vi "PQ_Windowed RMS.vi"(10 "data":waveform(dbl)[](array[waveform])) -> (1 "Resampled Data":dbl[][](graph), 2 "RMS":dbl[][](graph))   [LabVIEW 2014]
uses:
  <vilib>/Analysis/2dsp.llb/Rational Resample (multi-channel, DBL).vi
  <vilib>/imath/engines/lvmath2/RunTimeEngine/BuiltInFunctions/length/NIMS_length(GV).vi
  <instcachedir>/0/NIMS_length(GV)_08A3D13377FD4E4B96F5795FBF3698FA.lvgen/NIMS_length(GV)_08A3D13377FD4E4B96F5795FBF3698FA_000.vi
  <vilib>/imath/engines/lvmath2/RunTimeEngine/CommandStatement/MC_CommandStatement_break.vi
  <vilib>/imath/engines/lvmath2/RunTimeEngine/RangeToken/NIMS_Range.vi
  <instcachedir>/0/NIMS_Range_9BCE657718DF4976A877346C61F22738.lvgen/NIMS_Range_9BCE657718DF4976A877346C61F22738_000.vi
  <vilib>/imathl/engines/lvmath/Functions/Error Handling/Create Error.vi
  <vilib>/imath/engines/lvmath2/RunTimeEngine/VariableToken/NIMS_VariableToken_CondDefinedDefinedByReplace.vi
  <instcachedir>/0/NIMS_VariableToken_CondDefinedDefinedByReplace_D162CFFC24174562A9FEA619A91E1A56.lvgen/NIMS_VariableToken_CondDefinedDefinedByReplace_D162CFFC24174562A9FEA619A91E1A56_000.vi
  <vilib>/imath/engines/lvmath2/RunTimeSupport/NIMS_Error if Not Equal.vi
  <instcachedir>/0/NIMS_Error if Not Equal_8A0E9F659B9142D69417CC259581C4FD.lvgen/NIMS_Error if Not Equal_8A0E9F659B9142D69417CC259581C4FD_000.vi
  <instcachedir>/0/NIMS_Error if Not Equal_8A0E9F659B9142D69417CC259581C4FD.lvgen/NIMS_Error if Not Equal_8A0E9F659B9142D69417CC259581C4FD_001.vi
  <vilib>/imath/engines/lvmath2/RunTimeEngine/IndexRead/NIMS V(V).vi
  <instcachedir>/0/NIMS V(V)_298D9CB7BFEB42B8BC8D9C3C28AE8C70.lvgen/NIMS V(V)_298D9CB7BFEB42B8BC8D9C3C28AE8C70_000.vi
  <vilib>/imath/engines/lvmath2/RunTimeEngine/BuiltInFunctions/sum/NIMS_sum(GV).vi
  <instcachedir>/0/NIMS_sum(GV)_67F5EC36BC034E54A6BEC5B0673C00E5.lvgen/NIMS_sum(GV)_67F5EC36BC034E54A6BEC5B0673C00E5_000.vi
  <vilib>/imath/engines/lvmath2/RunTimeEngine/IndexReplace/NIMS V(S)=S.vi
  <instcachedir>/0/NIMS V(S)=S_2D52C4EC15D8415E870AEE69FB516CCA.lvgen/NIMS V(S)=S_2D52C4EC15D8415E870AEE69FB516CCA_001.vi
  <vilib>/imath/engines/lvmath2/RunTimeEngine/ErrorHandling/NIMS_Create Error From Enums.vi
  <vilib>/imath/engines/lvmath2/RunTimeEngine/CommandStatement/NIMS_CommandStatement_MaskErr.vi
  <vilib>/imath/engines/lvmath2/RunTimeEngine/VariableToken/NIMS_VariableToken_CondDefined.vi
  <instcachedir>/0/NIMS_VariableToken_CondDefined_EE8DD211A89249938CE6537267F5C9B3.lvgen/NIMS_VariableToken_CondDefined_EE8DD211A89249938CE6537267F5C9B3_000.vi
  <vilib>/imath/engines/lvmath2/RunTimeEngine/BuiltInFunctions/ones/NIMS_V=ones(I32,I32).vi
  <vilib>/imath/engines/lvmath2/RunTimeEngine/IndexRead/NIMS V(S).vi
  <instcachedir>/0/NIMS V(S)_0488751826AF41519A22953C041130DC.lvgen/NIMS V(S)_0488751826AF41519A22953C041130DC_003.vi
  <vilib>/imath/engines/lvmath2/RunTimeEngine/IndexReplace/NIMS V(V)=V.vi
  <instcachedir>/0/NIMS V(V)=V_1E3A7F7F615C46EF9FDD71F29C66FCF8.lvgen/NIMS V(V)=V_1E3A7F7F615C46EF9FDD71F29C66FCF8_000.vi
  <vilib>/imath/engines/lvmath2/RunTimeEngine/NodeEndStatement/NIMS_NodeEndStatement_Output.vi
  <instcachedir>/0/NIMS_NodeEndStatement_Output_53EC0D466D134D7ABD903AC30B43404B.lvgen/NIMS_NodeEndStatement_Output_53EC0D466D134D7ABD903AC30B43404B_005.vi
  <instcachedir>/0/NIMS_NodeEndStatement_Output_53EC0D466D134D7ABD903AC30B43404B.lvgen/NIMS_NodeEndStatement_Output_53EC0D466D134D7ABD903AC30B43404B_000.vi
  <vilib>/imath/engines/lvmath2/RunTimeEngine/ErrorHandling/NIMS_Finalize Error.vi
  <vilib>/Analysis/NI_AALPro.lvlib
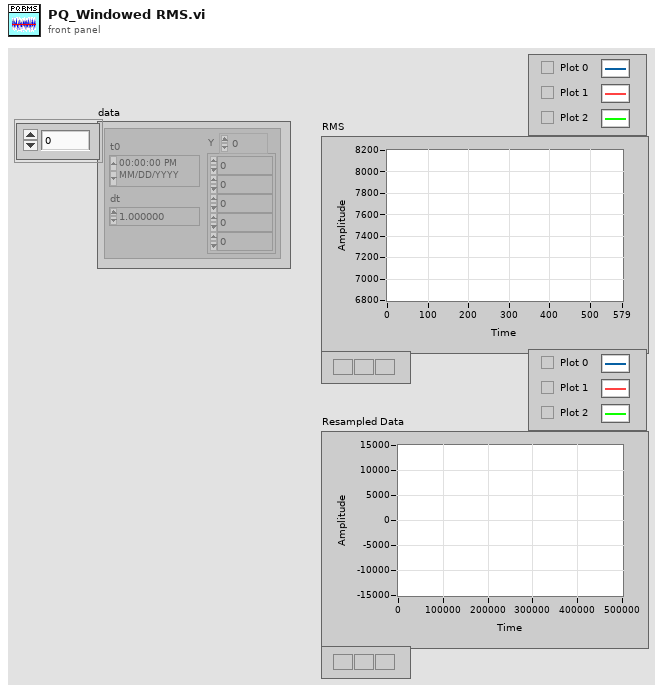
[diagram p1: front panel]
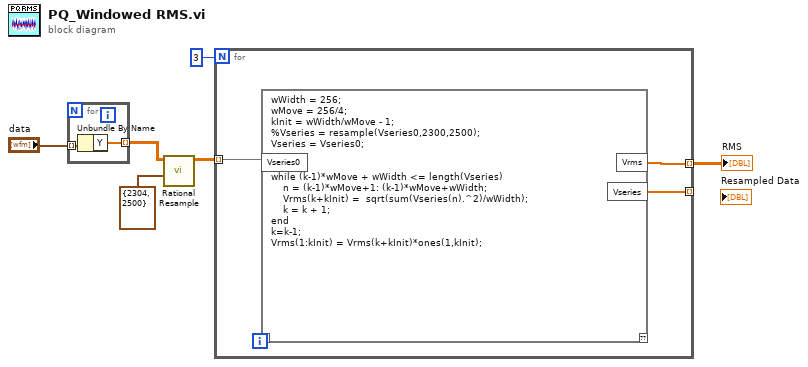
[diagram p0: block diagram]
diagram:
  n1 = for {
    tunnel: "data" -> [w8] mode=indexing
    tunnel: [w7] -> w1 mode=indexing
    n2 = Unbundle By Name(w8) -> ("Y"=w7:dbl[])
  }
  n3 = call-poly <vilib>:"Rational Resample.vi"("resample factor"=cluster{"interpolation":i32, "decimation":i32} {"interpolation"=2304, "decimation"=2500}, "X"=w1) -> ("Y"=w3:dbl[][])  [unwired: 7 in, 2 out]
  n4 = for {
    N: 3 -> [_]
    tunnel: [w11] -> _ mode=indexing
    tunnel: [w10] -> w6 mode=indexing
    tunnel: w3 -> [w9] mode=indexing
    n5 = mathscript code="wWidth = 256;\nwMove = 256/4;\nkInit = wWidth/wMove - 1;\n%Vseries = resample(Vseries0,2300,2500);\nVseries = Vseries0;\n \nk = 1;\nwhile (k-1)*wMove + wWidth <= length(Vseries)\n    n = (k-1)*wMove+1: (k-1)*wMove+wWidth;\n    Vrms(k+kInit) =  sqrt(sum(Vseries(n).^2)/wWidth);\n    k = k + 1;\nend\nk=k-1;\nVrms(1:kInit) = Vrms(k+kInit)*ones(1,kInit);"("Vseries0"=w9) -> ("Vrms"=w10:cdb[], "Vseries"=w11:dbl[])  [unwired: 1 in, 1 out]
  }
  "RMS" <- w6
